vi "sendValue.vi"(8 "error in (no error)":errorcluster, 10 "data":variant, 11 "setDigitalFilter in":refnum<class "setDigitalFilter.lvclass">) -> (0 "error out":errorcluster, 2 "function return":i32, 3 "setDigitalFilter out":refnum<class "setDigitalFilter.lvclass">)   [LabVIEW 2016, in "SALLV_MtAtElectrometer_Messaging.lvlib" / "setDigitalFilter.lvclass"]
uses:
  setDigitalFilter.lvclass
  ts_sallv_MtAtElectrometer/DataTypes/command_setDigitalFilter.ctl
  ts_sallv_MtAtElectrometer/SALLV_MtAtElectrometer.lvlib
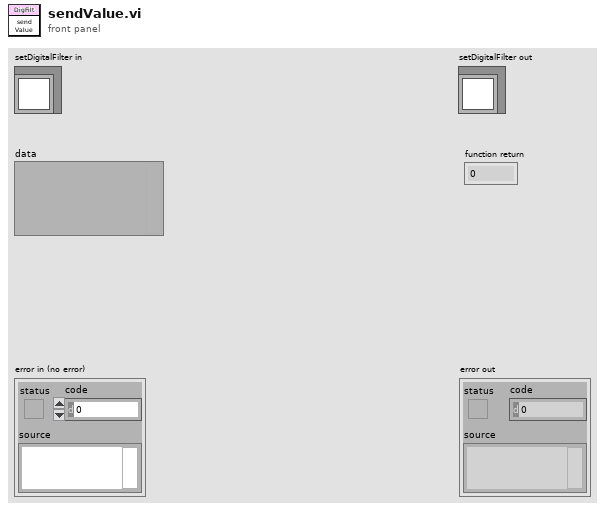
[diagram p1: front panel]
types:
  T1 = typedef "SALLV_MtAtElectrometer.lvlib/command_setDigitalFilter.ctl" = cluster{"activateFilter":bool, "averageFilter":u16, "medianFilter":bool}
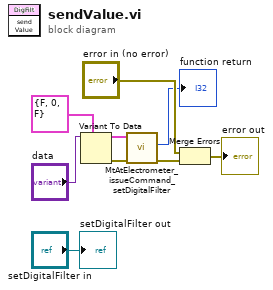
[diagram p0: block diagram]
diagram:
  n1 = Variant To Data(type=T1 {"activateFilter"=FALSE, "averageFilter"=0, "medianFilter"=FALSE} ("command_setDigitalFilter_Ctl"), Variant="data") -> (data=w3:T1, error out=w4:errorcluster)  [unwired: 1 in]
  n2 = call "MtAtElectrometer_issueCommand_setDigitalFilter.vi"("error in (no error)"=w4, "command_setDigitalFilter_Ctl"=w3) -> ("error out"=w5:errorcluster, "function return"=→"function return":i32)  [unwired: 7 in, 1 out]
  n3 = Merge Errors("error in (no error)", w5) -> (→"error out":errorcluster)
  "setDigitalFilter out" <- "setDigitalFilter in"
